vi "Settings - NI 9472.vi"(8 "Error In":errorcluster) -> (0 "Error Out":errorcluster={"status"=TRUE, "code"=-200077, "source"="Property Node DAQmx Channel (arg 2) in DAQmx Create Channel (AI-Temperature-Thermocouple).vi:1->Settings - NI 9211.vi <append>\n<B>Property: </B>AI.Temp.Units\n<B>Requested Value: </B>\n<B>You Can Select: </B>Deg C, Deg F, Kelvins, Deg R, From Custom Scale\n\n<B>Channel Name: </B>Temperature\n\n<B>Task Name: </B>_unnamedTask<E>"}, 3 "Cancelled?":bool)   [LabVIEW 2011]
doc: "This VI will get settings for NI 9211 measurement."
uses:
  SubVIs/Controls/TransparencyEffectOperations.ctl
  <vilib>/DAQmx/write.llb/DAQmx Write.vi
  <vilib>/DAQmx/write.llb/DAQmx Write (Digital 1D U8 NChan 1Samp).vi
  <vilib>/DAQmx/create/channels.llb/DAQmx Create Channel (DO-Digital Output).vi
  <vilib>/DAQmx/miscellaneous.llb/DAQmx Fill In Error Info.vi
  Program Files/National Instruments/LabVIEW 2011/resource/objmgr/daqmx.rc
panel:
  out "DIO Leds":bool[](array[boolean])
  in  "DIO States":bool[](array[boolean])=[FALSE, FALSE, FALSE, FALSE, FALSE, FALSE, FALSE, FALSE]
  in  "Invert Lines?":bool
  in  "Header For Measurement File":string="Temperature CH0"
  in  "Cancel Button":bool
  in  "OK Button":bool
  # "NI 9472"
  # "Meas File Settings"
  # "Hardware Settings"
  # "Initial State"
  # "on"
  # "on"
  # "off"
  # "off"
  # "0   1   2   3   4   5   6   7"
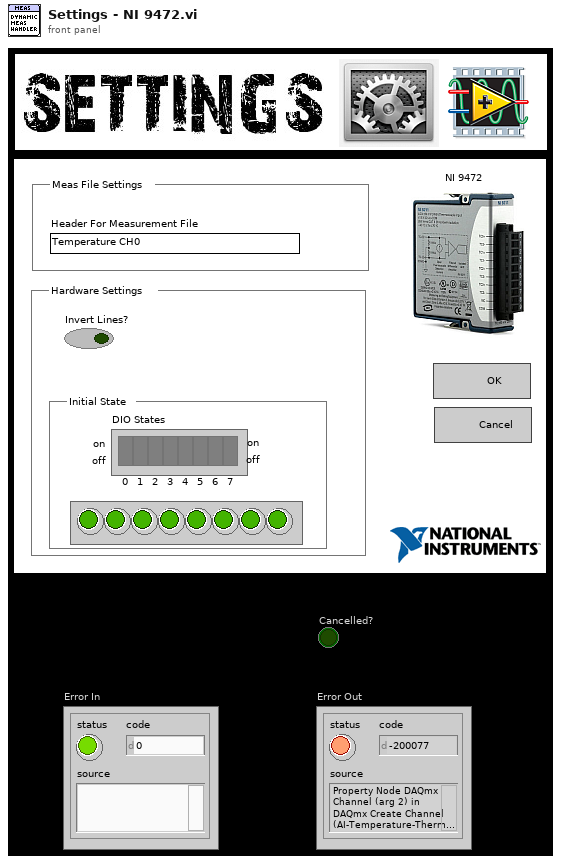
[diagram p1: front panel]
types:
  T1 = typedef "TransparencyEffectOperations.ctl" = enum16{"Show", "Hide 80%", "Hide All"}
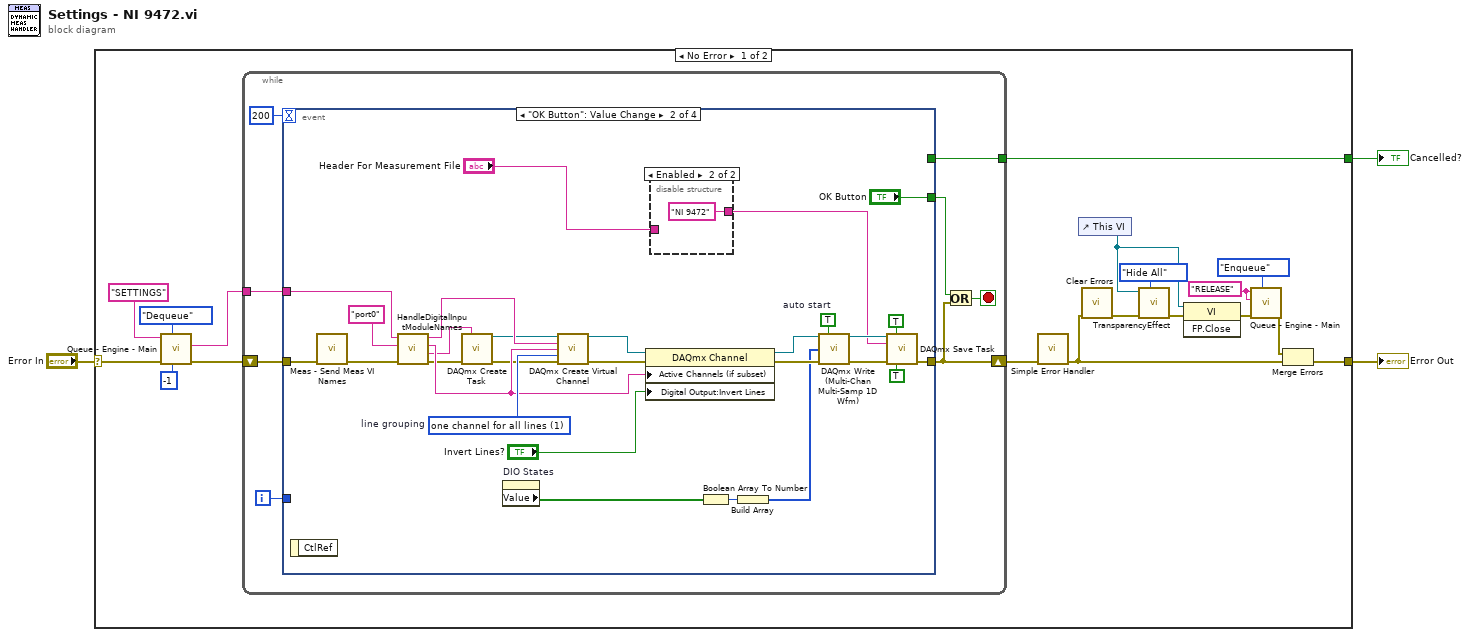
[diagram p0: block diagram]
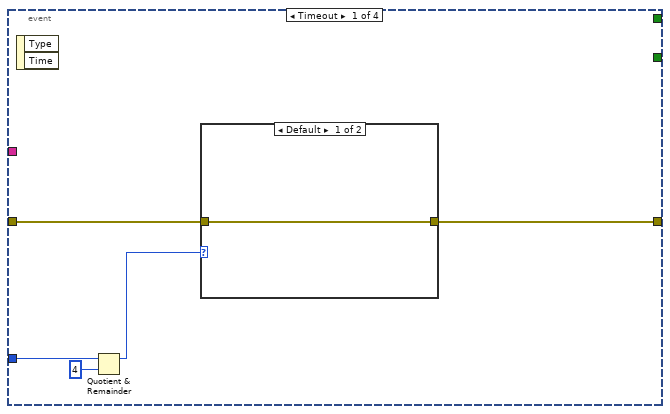
[diagram p2: hidden frame]
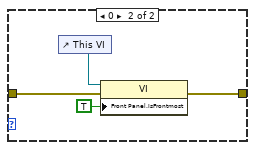
[diagram p3: hidden frame]
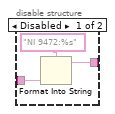
[diagram p4: hidden frame]
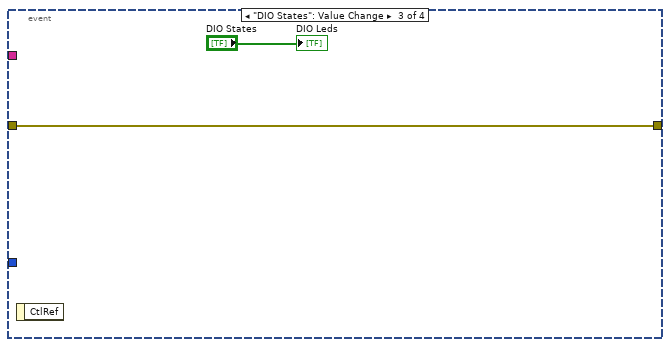
[diagram p5: hidden frame]
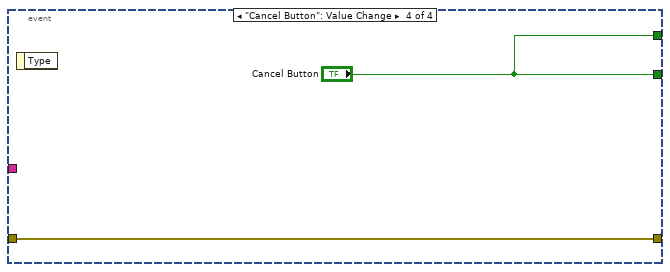
[diagram p6: hidden frame]
diagram:
  n1 = case shown="No Error" "Error In" {
    selector: "Error In" -> [w18 w76]
    tunnel: [w21 _] -> w3
    tunnel: [w4 w76] -> w2
    frame No Error {
      w10 = "RELEASE" ("Queue Data In")
      n2 = call "Queue - Engine - Main.vi"("timeout in ms (-1)"=-1, "Operation"=enum16{"Enqueue", "Dequeue", "Flush", "Release"}."Dequeue", "error in"=w18, "Queue Name In"="SETTINGS") -> ("error out"=w17:errorcluster, "Data Out"=w16:string)  [unwired: 5 in, 1 out]
      n3 = while {
        tunnel: [w29] -> w21
        shift-right: [w24] -> w5
        shift-left: w17 -> [w28]
        tunnel: w16 -> [w27]
        i -> [w25]
        stop <- w22 stop-if-true
        n4 = event shown="[1] \"OK Button\": Value Change" {
          selector: _ -> [_ _ _ _]
          dyn-events: _ -> [_ _ _ _]
          timeout: 200 -> [_ _ _ _]
          tunnel: [_ "OK Button" _ "Cancel Button"] -> w23
          tunnel: [_ _ _ "Cancel Button"] -> w29
          tunnel: [w33 w42 w72 w74] -> w24
          tunnel: w28 -> [w34 w64 w72 w74]
          tunnel: w27 -> [_ w66 _ _]
          tunnel: w25 -> [w32 _ _ _]
          event Timeout {
            n5 = event-data() -> ()  [unwired: 1 in, 2 out]
            n6 = Quotient & Remainder(x=w32, y=4) -> (x-y*floor(x/y)=w30:i32)  [unwired: 1 out]
            n7 = case shown="Default" w30 {
              tunnel: w34 -> [w35 w38]
              tunnel: [w35 w37] -> w33
              frame Default {
              }
              frame 0 {
                n8 = control-ref of="This VI"() -> (w39:refnum<vi>)
                n9 = property class="VI"(reference=w39, error in=w38, "Front Panel.IsFrontmost"=TRUE ("Front Panel Window:Is Frontmost")) -> (error out=w37:errorcluster)  [unwired: 1 out]
              }
            }
          }
          event "OK Button": Value Change {
            w58 = TRUE  # auto start
            w60 = 1 items=["one channel for each line", "one channel for all lines"]  # line grouping
            n10 = event-data() -> ()  [unwired: 1 in, 1 out]
            n11 = call "Meas - Send Meas VI Names.vi"("Error In"=w64) -> ("Error Out"=w63:errorcluster)  [unwired: 10 in]
            n12 = call "HandleDigitalInputModuleNames.vi"("Error In"=w63, "Port Name In"="port0", "Data In"=w66) -> ("Error Out"=w50:errorcluster, "Meas Name"=w49:string, "Module and CH"=w59:string, "Channel"=w54:string)  [unwired: 5 in]
            n13 = call <vilib>:"DAQmx Create Task.vi"("new task name"=w49, "error in"=w50) -> ("task out"=w48:refnum<k21>, "error out"=w47:errorcluster)  [unwired: 3 in, 9 out]
            n14 = property on="DIO States" class="Arr (strict)"() -> ("Value"=w46:bool[])  [unwired: 2 in, 2 out]
            n15 = call-poly <vilib>:"DAQmx Create Virtual Channel.vi"("task in"=w48, "lines"=w54, "name to assign"=w59, "line grouping"=w60, "error in"=w47) -> ("task out"=w61:refnum<k21>, "error out"=w62:errorcluster)  [unwired: 9 out]
            n16 = property class="DAQmx Channel"(reference=w61, error in=w62, "Active Channels (if subset)"=w59, "Digital Output:Invert Lines"="Invert Lines?") -> (reference out=w56:refnum<k21>, error out=w57:errorcluster)
            n17 = disable-structure shown="Enabled" {
              disable-tunnel: "Header For Measurement File" -> [w69 _]
              disable-tunnel: [w68 "NI 9472" ("Variable In")] -> w40
              frame Disabled {
                n18 = Format Into String(format string="NI 9472:%s", w69) -> (resulting string=w68:string)  [unwired: 2 in, 1 out]
              }
              frame Enabled {
              }
            }
            n19 = Boolean Array To Number(Boolean array=w46) -> (number=w52:u32)
            n20 = Build Array(w52) -> (w51:u32[])
            n21 = call-poly "DAQmx Write (Multi-Chan Multi-Samp 1D Wfm).vi"("task/channels in"=w56, "auto start"=w58, "data"=w51, "error in"=w57) -> ("task out"=w41:refnum<k21>, "error out"=w43:errorcluster)  [unwired: 10 out]
            n22 = call <vilib>:"DAQmx Save Task.vi"("task/channels in"=w41, "allow interactive editing?"=TRUE, "save as"=w40, "error in"=w43, "overwrite existing task?"=TRUE) -> ("error out"=w42:errorcluster)  [unwired: 9 in, 1 out]
          }
          event "DIO States": Value Change {
            n23 = event-data() -> ()  [unwired: 1 in, 1 out]
            "DIO Leds" <- "DIO States"
          }
          event "Cancel Button": Value Change {
            n24 = event-data() -> ()  [unwired: 1 in, 1 out]
          }
        }
        n25 = Or(x=w23, y=w24) -> (x .or. y?=w22:bool)
      }
      n26 = call <vilib>:"Simple Error Handler.vi"("error in (no error)"=w5) -> ("error out"=w7:errorcluster)  [unwired: 4 in, 4 out]
      n27 = control-ref of="This VI"() -> (w14:refnum<vi>)
      n28 = call <vilib>:"Clear Errors.vi"("error in (no error)"=w7) -> ("error out"=w6:errorcluster)  [unwired: 6 in]
      n29 = call "TransparencyEffect.vi"("Operation"=TransparencyEffectOperations."Hide All", "error in"=w6, "VI Ref in"=w14) -> ("error out"=w11:errorcluster)  [unwired: 8 in]
      n30 = invoke class="VI" method="FP.Close"(reference=w14, error in=w11) -> (error out=w8:errorcluster)  [unwired: 1 in, 2 out]
      n31 = call "Queue - Engine - Main.vi"("Operation"=enum16{"Enqueue", "Dequeue", "Flush", "Release"}."Enqueue", "error in"=w8, "Queue Data In"=w10, "Queue Name In"=w10) -> ("error out"=w9:errorcluster)  [unwired: 5 in, 2 out]
      n32 = Merge Errors(w9, w7) -> (w4:errorcluster)
    }
    frame Error {
    }
  }
  "Cancelled?" <- w3
  "Error Out" <- w2
